vi "Save Config.vi"(8 "error in (no error)":errorcluster, 11 "Motion Controller in":refnum<class "FINE SIM Motion Axis.lvclass">) -> (0 "error out":errorcluster, 3 "Motion Controller out":refnum<class "FINE SIM Motion Axis.lvclass">)   [LabVIEW 2022 SP3, in "FINE SIM Motion Axis.lvclass"]
uses:
  FINE SIM Motion Axis.lvclass
  369b6a7b-23d0-449b-bf9f-668cb5c7d15f.vi
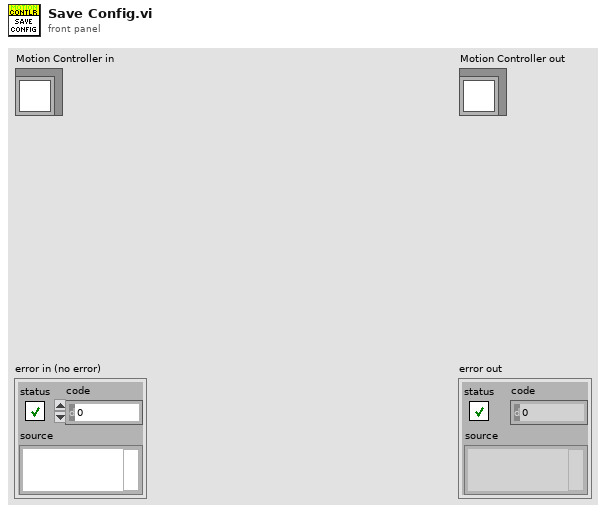
[diagram p1: front panel]
types:
  T1 = typedef "FINE SIM Motion Axis.lvclass/Axis Data.ctl" = cluster{"Axis Parameters":T2, "Time Stamp":timestamp, "Settings":T4}
  T2 = typedef "FINE SIM Motion Axis.lvclass/Axis Parameters.ctl" = cluster{"Moving":bool, "Homed":bool, "Desired Position":dbl, "Current Positon":dbl, "Current Speed":dbl, "Home Status":T3}
  T3 = typedef "FINE SIM Motion Axis.lvclass/Homing Status.ctl" = enum16{"Idle", "Inital Home Motion", "Final Home Motion", "Done Homing"}
  T4 = typedef "FINE SIM Motion Axis.lvclass/Settings.ctl" = cluster{"Axis Name":string, "Axis Settings":T5}
  T5 = typedef "FINE SIM Motion Axis.lvclass/Axis Settings.ctl" = cluster{"Speed":dbl, "Acceleration":dbl}
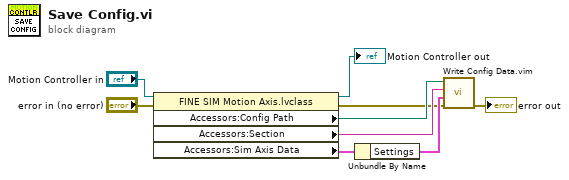
[diagram p0: block diagram]
diagram:
  n1 = property class="FINE SIM Motion Axis.lvclass"(reference="Motion Controller in", error in="error in (no error)") -> (reference out=→"Motion Controller out":refnum<class "FINE SIM Motion Axis.lvclass">, error out=w1:errorcluster, "Accessors:Config Path"=w7:path, "Accessors:Section"=w6:string, "Accessors:Sim Axis Data"=w5:T1)
  n2 = Unbundle By Name(w5) -> ("Settings"=w4:T4)
  n3 = call "Write Config Data.vim"("error in (no error)"=w1, "Section Formatted Cluster Type"=w4, "Section"=w6, "Config Path"=w7) -> ("error out"=→"error out":errorcluster)  [unwired: 7 in]
